vi "手动启动选择对话框.vi"() -> (2 "确定":bool, 3 "输出簇":cluster{"多参数":bool, "氨氮":bool, "CODcr":bool})   [LabVIEW 2016, in "PLC.lvlib"]
uses:
  PLC.lvlib
panel:
  in  "氨氮":bool
  in  "CODcr":bool
  in  "多参数":bool
  in  "取消":bool
  in  "确定":bool
  # "请选择启动参数"
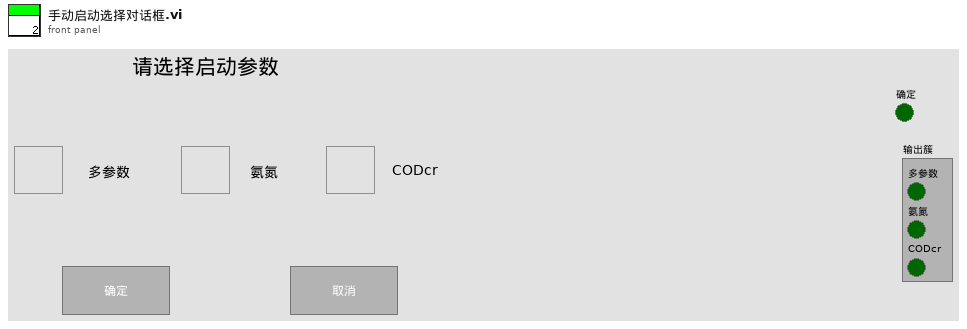
[diagram p1: front panel]
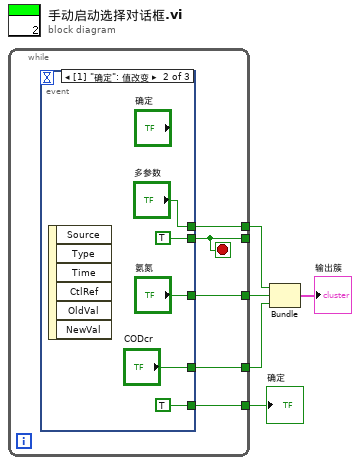
[diagram p0: block diagram]
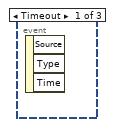
[diagram p2: hidden frame]
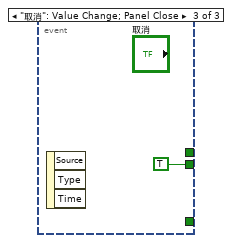
[diagram p3: hidden frame]
diagram:
  n1 = while {
    tunnel: [w10] -> w5
    tunnel: [w9] -> w4
    tunnel: [w8] -> w3
    tunnel: [w7] -> _
    tunnel: [w6] -> w1
    stop <- w7 stop-if-true
    n2 = event shown="[1] \"确定\": 值改变" {
      selector: _ -> [_ _ _]
      dyn-events: _ -> [_ _ _]
      timeout: _ -> [_ _ _]
      tunnel: [_ TRUE TRUE] -> w7
      tunnel: [_ "多参数" _] -> w10
      tunnel: [_ "氨氮" _] -> w9
      tunnel: [_ "CODcr" _] -> w8
      tunnel: [_ TRUE _] -> w6
      event Timeout {
        n3 = event-data() -> ()  [unwired: 1 in, 3 out]
      }
      event "确定": Value Change {
        n4 = event-data() -> ()  [unwired: 1 in, 6 out]
      }
      event "取消": Value Change; Panel Close {
        n5 = event-data() -> ()  [unwired: 1 in, 3 out]
      }
    }
  }
  "确定" <- w1
  n6 = Bundle("多参数"=w5, "氨氮"=w4, "CODcr"=w3) -> (→"输出簇":cluster{"多参数":bool, "氨氮":bool, "CODcr":bool})  [unwired: 1 in]
